vi "Gaussian_Rolloff_Dialog.vi"() -> (2 "Rolloff (dB) 2":dbl=3.0 min=1.0 max=10.0, 3 "Cancelled?":bool)   [LabVIEW 2015]
doc: "Shows current profiles on the box for selection."
panel:
  in  "Rolloff (dB)":dbl=3.0 min=1.0 max=10.0
  in  "Cancel":bool
  in  "OK":bool
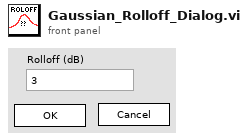
[diagram p1: front panel]
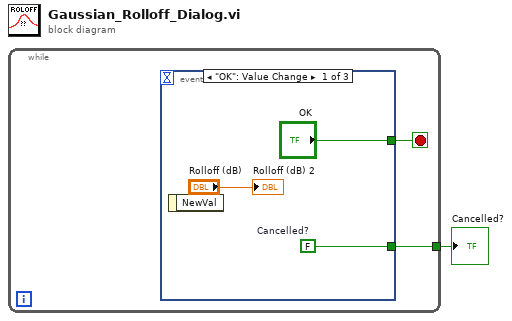
[diagram p0: block diagram]
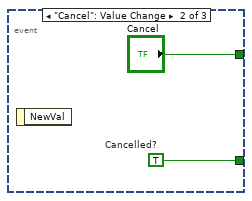
[diagram p2: hidden frame]
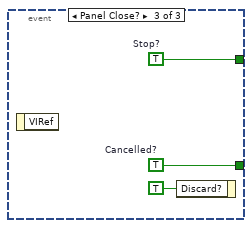
[diagram p3: hidden frame]
diagram:
  n1 = while {
    tunnel: [w2] -> w1
    stop <- w3 stop-if-true
    n2 = event shown="[0] \"OK\": Value Change" {
      selector: _ -> [_ _ _]
      dyn-events: _ -> [_ _ _]
      timeout: _ -> [_ _ _]
      tunnel: ["OK" "Cancel" w10] -> w3
      tunnel: [w6 w8 w9] -> w2
      event "OK": Value Change {
        w6 = FALSE  # Cancelled?
        n3 = event-data() -> ()  [unwired: 1 in, 1 out]
        "Rolloff (dB) 2" <- "Rolloff (dB)"
      }
      event "Cancel": Value Change {
        w8 = TRUE  # Cancelled?
        n4 = event-data() -> ()  [unwired: 1 in, 1 out]
      }
      event Panel Close? {
        w9 = TRUE  # Cancelled?
        w10 = TRUE  # Stop?
        n5 = event-data() -> ()  [unwired: 1 in, 1 out]
        n6 = event-data("Discard?"=TRUE) -> ()  [unwired: 1 in, 1 out]
      }
    }
  }
  "Cancelled?" <- w1
